vi "Phase_Step_Transfer.vi"(11 "Input_Phase_Step":i32) -> (3 "Output_Phase_Step":i32)   [LabVIEW 2023, in "ELTA.lvlib"]
uses:
  ELTA.lvlib
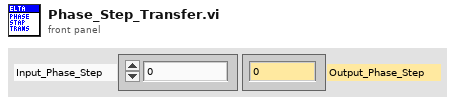
[diagram p1: front panel]
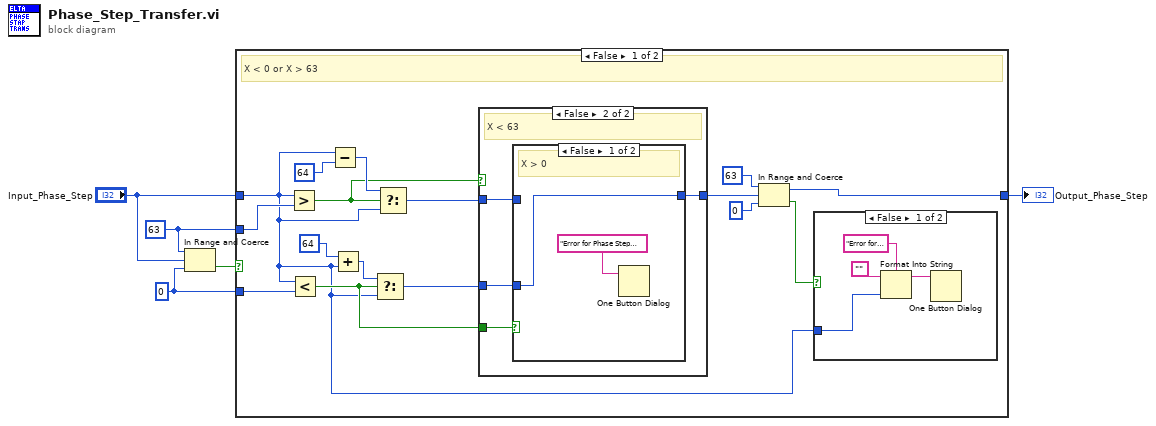
[diagram p0: block diagram]
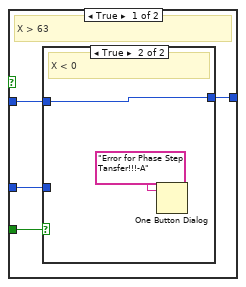
[diagram p3: hidden frame]
diagram:
  w2 = 0 ("lower limit")
  w3 = 63 ("upper limit")
  n1 = In Range and Coerce(upper limit=w3, x="Input_Phase_Step", lower limit=w2) -> (In Range?=w5:bool)  [unwired: 1 out]
  n2 = case shown="False" w5 {
    tunnel: "Input_Phase_Step" -> [w6 w40]
    tunnel: [w7 w40] -> w4
    tunnel: w3 -> [w21 _]
    tunnel: w2 -> [w20 _]
    frame False {
      # "X < 0 or X > 63"
      n3 = Greater?(x=w6, y=w21) -> (0:w15:bool)
      n4 = Less?(x=w6, y=w20) -> (x < y?=w13:bool)
      n5 = Subtract(x=w6, y=64) -> (x-y=w18:i32)
      n6 = Add(x=64, y=w6) -> (x+y=w16:i32)
      n7 = Select(t=w16, s=w13, f=w6) -> (s? t:f=w14:i32)
      n8 = Select(t=w18, s=w15, f=w6) -> (s? t:f=w12:i32)
      n9 = case shown="False" w15 {
        tunnel: w14 -> [w27 w34]
        tunnel: w13 -> [w29 w36]
        tunnel: w12 -> [w28 w35]
        tunnel: [w26 w33] -> w11
        frame True {
          # "X > 63"
          n10 = case shown="True" w29 {
            tunnel: w28 -> [w30 w31]
            tunnel: w27 -> [_ _]
            tunnel: [w30 w31] -> w26
            frame False {
              # "X > 0"
            }
            frame True {
              # "X < 0"
              n11 = One Button Dialog(message="Error for Phase Step Tansfer!!!-A") -> ()  [unwired: 1 in, 1 out]
            }
          }
        }
        frame False {
          # "X < 63"
          n12 = case shown="False" w36 {
            tunnel: w35 -> [_ _]
            tunnel: w34 -> [w38 w39]
            tunnel: [w38 w39] -> w33
            frame False {
              # "X > 0"
              n13 = One Button Dialog(message="Error for Phase Step Tansfer!! -B") -> ()  [unwired: 1 in, 1 out]
            }
            frame True {
              # "X < 0"
            }
          }
        }
      }
      n14 = In Range and Coerce(upper limit=63, x=w11, lower limit=0) -> (coerced(x)=w7:i32, In Range?=w8:bool)
      n15 = case shown="False" w8 {
        tunnel: w6 -> [w23 _]
        frame False {
          n16 = Format Into String(format string="Error for Phase Step Tansfer!!\nOver Step : [%d]" ("message"), initial string="", w23) -> (resulting string=w22:string)  [unwired: 1 in, 1 out]
          n17 = One Button Dialog(message=w22) -> ()  [unwired: 1 in, 1 out]
        }
        frame True {
        }
      }
    }
    frame True {
      # "0 <= X <= 63"
    }
  }
  "Output_Phase_Step" <- w4
